vi "Write Data.vi"(8 "error in (no error)":errorcluster, 9 "Publication Time":timestamp, 10 "Value":variant, 11 "QueueTransport In":refnum<class "QueueTransport.lvclass">) -> (0 "error out":errorcluster, 3 "QueueTransport Out":refnum<class "QueueTransport.lvclass">)   [LabVIEW 2019, in "QueueTransport.lvclass"]
doc: "<License>\nCopyright © 2017 Composed Systems, LLC | All rights reserved\nwww.composed.io\n\nAuthor: Ethan Stern <ethan.stern@composed.io>\n\nThis software is provided \"AS IS\" WITHOUT WARRANTIES, either express or implied, AND IS FOR EDUCATIONAL PURPOSES ONLY.\n</License>"
uses:
  <vilib>/gpm_packages/@cs/transport/Source/Concrete/QueueTransport/QueueTransport.lvclass
  <vilib>/gpm_packages/@cs/transport/Source/Concrete/QueueTransport/QueueTransport.lvclass/QueueTransport.ctl
  <vilib>/Utility/error.llb/Error Cluster From Error Code.vi
  <vilib>/ErrorRing/Error Ring.xnode
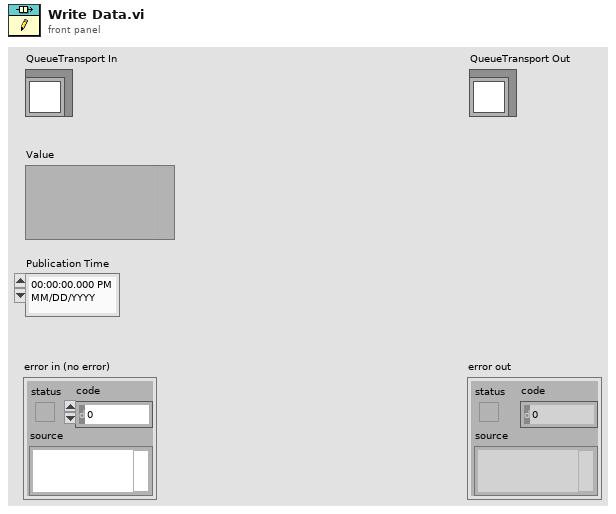
[diagram p1: front panel]
types:
  T1 = cluster{"Value":variant, "Publication Time":timestamp}
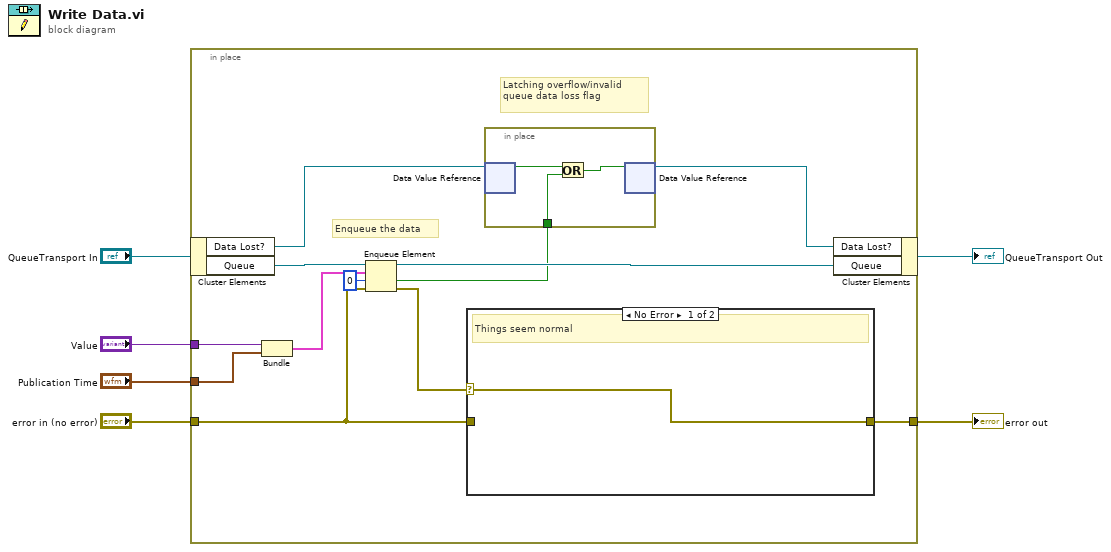
[diagram p0: block diagram]
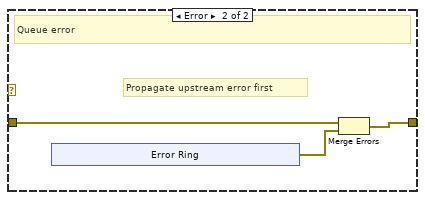
[diagram p2: hidden frame]
diagram:
  n1 = in-place {
    in-place-border: "error in (no error)" -> [w9]
    in-place-border: "Value" -> [w18]
    in-place-border: "Publication Time" -> [w17]
    in-place-border: [w12] -> w1
    # "Latching overflow/invalid\nqueue data loss flag"
    # "Enqueue the data"
    n2 = in-place-cluster #1("QueueTransport In") -> ("Data Lost?"=w8:refnum<data-value>, "Queue"=w15:refnum<queue>)
    n3 = Bundle("Value"=w18, "Publication Time"=w17) -> (w16:T1)  [unwired: 1 in]
    n4 = Enqueue Element(queue=w15, element=w16, timeout in ms (-1)=0, error in (no error)=w9) -> (queue out=w14:refnum<queue>, timed out?=w10:bool, error out=w13:errorcluster)
    n5 = case shown="No Error" w13 {
      selector: w13 -> [w22 _]
      tunnel: [w22 w25] -> w12
      tunnel: w9 -> [_ w23]
      frame No Error {
        # "Things seem normal"
      }
      frame Error {
        # "Propagate upstream error first"
        # "Queue error"
        n6 = xnode "Error Ring"() -> ("error out"=w24:errorcluster)
        n7 = Merge Errors(w23, w24) -> (w25:errorcluster)
      }
    }
    n8 = in-place {
      in-place-border: w10 -> [w21]
      n9 = in-place-dvr #2(w8) -> (w20:bool)  [unwired: 1 out]
      n10 = Or(x=w20, y=w21) -> (x .or. y?=w19:bool)
      n11 = in-place-dvr #2(w19) -> (w7:refnum<data-value>)  [unwired: 1 out]
    }
    n12 = in-place-cluster #1("Data Lost?"=w7, "Queue"=w14) -> (→"QueueTransport Out":refnum<class "QueueTransport.lvclass">)
  }
  "error out" <- w1
